vi "task6_BINARY2DEC_CONVERTER_LOGGING_OUTPUT.vi"() -> ()   [LabVIEW 2017]
uses:
  <vilib>/Platform/TimedLoop/XDataNode/timing_clust.ctl
  <vilib>/Platform/TimedLoop/XDataNode/nitl_modes.ctl
  <vilib>/Platform/TimedLoop/XDataNode/wakeup.ctl
  <vilib>/platform/TimedLoop/XDataNode/XDataNode.xnode
  <vilib>/Platform/TimedLoop/XDataNode/XDNodeRunTimeDep.lvlib
panel:
  out "Waveform Chart":i16(graph)
  out "display":dbl
  in  "2^0":bool
  in  "2^1":bool
  in  "2^2":bool
  in  "2^3":bool
  in  "2^4":bool
  in  "2^5":bool
  in  "2^6":bool
  in  "2^7":bool
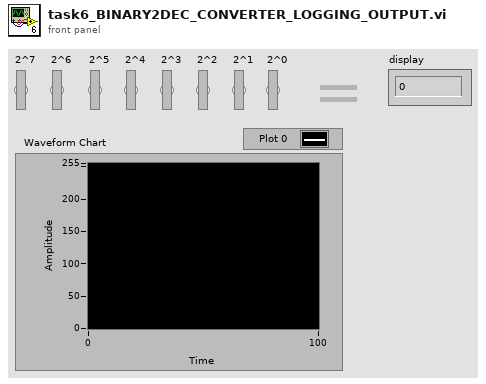
[diagram p1: front panel]
types:
  T1 = typedef "XDNodeRunTimeDep.lvlib/timing_clust.ctl" = cluster{"Expected End [f-1]":u64, "Actual End [f-1]":u64, "Finished Late? [f-1]":bool, "Expected End [i-1]":u64, "Actual End [i-1]":u64, "Finished Late? [i-1]":bool, "Expected Start [i]":u64, "Actual Start [i]":u64, "Expected Start [f]":u64, "Actual Start [f]":u64, "Source Name":string, "Structure Name":string, "Period":i64, "Deadline":i64, "Offset":i64, "Start":i64, "Priority":i32, "Timeout":i32, "Mode":T2, "Wakeup Reason":T3, "Error":errorcluster, "Source Type":string, "Secondary Source Type":string, "Global End Time":u64, "Global Start Time":u64, "Frame Duration":u64, "Iteration Duration":u64, "Assigned CPU":i32, "I/O Scan Engine Mode":u32}
  T2 = typedef "XDNodeRunTimeDep.lvlib/nitl_modes.ctl" = enum32{"No Change", "Process missed periods, maintain original phase", "Discard missed periods, maintain original phase", "Process missed periods, ignore original phase", "Discard missed periods, ignore original phase"}
  T3 = typedef "XDNodeRunTimeDep.lvlib/wakeup.ctl" = enum32{"Normal", "Aborted", "Asynchronous wakeup", "Timing source error", "Timed loop error", "Timeout"}
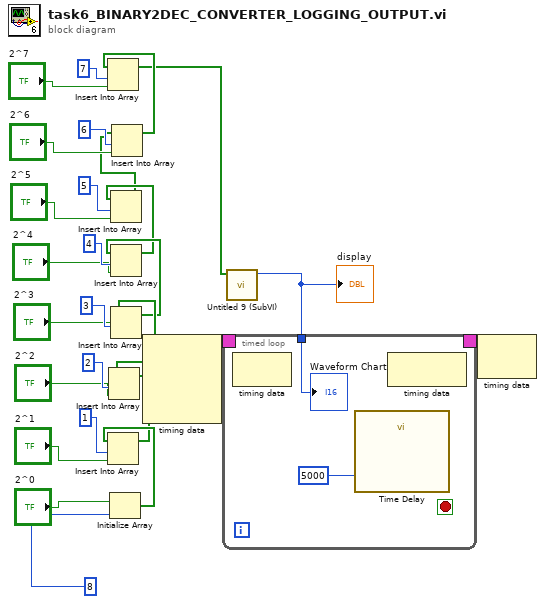
[diagram p0: block diagram]
diagram:
  n1 = Initialize Array("2^0", 8) -> (w11:bool[])
  n2 = Insert Into Array(array=w11, index=1, new element="2^1") -> (w10:bool[])
  n3 = Insert Into Array(array=w10, index=2, new element="2^2") -> (w9:bool[])
  n4 = Insert Into Array(array=w9, index=3, new element="2^3") -> (w8:bool[])
  n5 = Insert Into Array(array=w8, index=4, new element="2^4") -> (w7:bool[])
  n6 = Insert Into Array(array=w7, index=5, new element="2^5") -> (w6:bool[])
  n7 = Insert Into Array(array=w6, index=6, new element="2^6") -> (w5:bool[])
  n8 = Insert Into Array(array=w5, index=7, new element="2^7") -> (w4:bool[])
  n9 = node-c288() -> (w3:T1)  [unwired: 4 in]
  n10 = call "Untitled 9 (SubVI).vi"("Array"=w4) -> ("Numeric"=w1:i16)  [unwired: 10 in]
  "display" <- w1
  n11 = timed-loop {
    timing: w3 -> [_]
    timing-out: [_] -> w2
    tunnel: w1 -> [w29]
    stop <- _ stop-if-true
    n12 = node-c288() -> ()  [unwired: 1 in, 1 out]
    n13 = call "Time Delay"("Delay Time (s)"=5000) -> ()  [unwired: 10 in, 1 out]
    n14 = node-c288() -> ()  [unwired: 1 in, 1 out]
    "Waveform Chart" <- w29
  }
  n15 = node-c288(w2) -> ()  [unwired: 1 out]
